vi "Configure Data Buffer.vi"(0 "VISA resource name":refnum<visa-resource-name>, 1 "Buffer Size (1000)":i32=1000, 5 "Enable Buffer Auto Clear (True)":bool=TRUE, 7 "Source (0: Measurement Data)":u16(ring) items=["Measurement Data", "Math Data", "None"], 9 "Buffer Control Mode (2: Always)":u16(ring)=2 items=["Never", "Next", "Always"], 11 "error in (no error)":errorcluster, 12 "Relative Timestamp Format (0:ABS)":u16(ring) items=["Absolute", "Delta"]) -> (4 "VISA resource name out":refnum<visa-resource-name>, 15 "error out":errorcluster)   [LabVIEW 2020, in "Keithley 27XX.lvlib"]
doc: "This VI allows you to control the Data Store. It controls the size of the buffer, the source of the data, and other controls on the data buffer."
uses:
  <instrlib>/Keithley 27XX/Keithley 27XX.lvlib
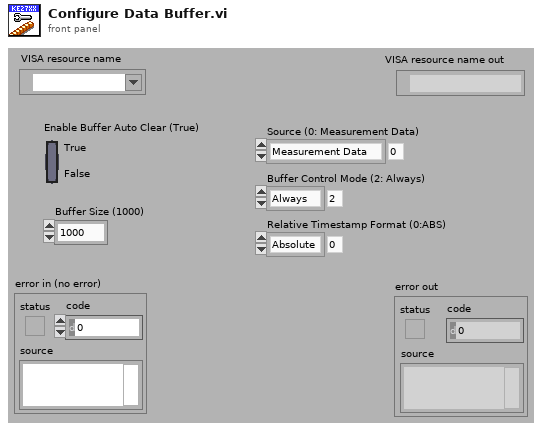
[diagram p1: front panel]
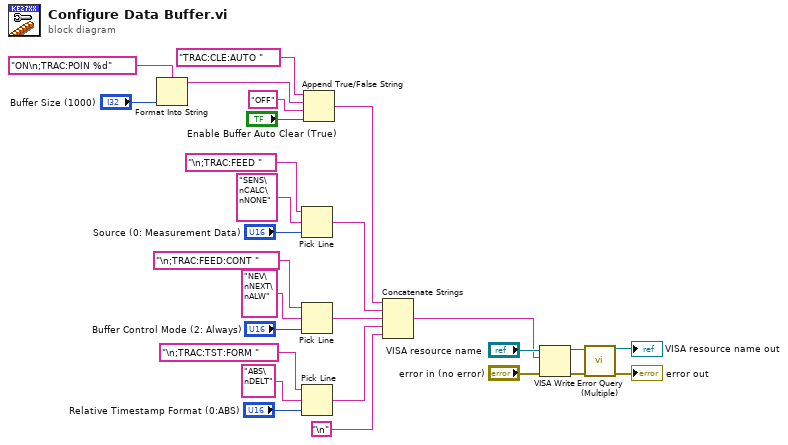
[diagram p0: block diagram]
diagram:
  n1 = Format Into String(format string="ON\n;TRAC:POIN %d", "Buffer Size (1000)") -> (resulting string=w3:string)  [unwired: 2 in, 1 out]
  n2 = Pick Line(string ("")="\n;TRAC:FEED ", multi-line string="SENS\nCALC\nNONE", line index="Source (0: Measurement Data)") -> (output string=w17:string)
  n3 = Pick Line(string ("")="\n;TRAC:FEED:CONT ", multi-line string="NEV\nNEXT\nALW", line index="Buffer Control Mode (2: Always)") -> (output string=w16:string)
  n4 = Pick Line(string ("")="\n;TRAC:TST:FORM ", multi-line string="ABS\nDELT", line index="Relative Timestamp Format (0:ABS)") -> (output string=w2:string)
  n5 = Append True/False String(1:"Enable Buffer Auto Clear (True)", 2:"OFF" ("false string"), 3:w3, 4:"TRAC:CLE:AUTO " ("false string")) -> (0:w18:string)
  n6 = Concatenate Strings(w18, w17, w16, w2, "\n") -> (w13:string)
  n7 = VISA Write(VISA resource name="VISA resource name", write buffer=w13, error in (no error)="error in (no error)") -> (VISA resource name out=w7:refnum<visa-resource-name>, error out=w6:errorcluster)  [unwired: 1 out]
  n8 = call <instrlib>:"Error Query (Multiple).vi"("VISA resource name"=w7, "error in (no error)"=w6) -> ("VISA resource name out"=→"VISA resource name out":refnum<visa-resource-name>, "error out"=→"error out":errorcluster)  [unwired: 10 in, 2 out]
